vi "StatusPub0MQ.vi"() -> (0 "error":errorcluster)   [LabVIEW 2018]
uses:
  <vilib>/addons/zeromq/zmq_context.lvclass
  <vilib>/addons/zeromq/zmq_socket.lvclass
  <vilib>/addons/zeromq/socket_type.ctl
  Global_Telescopio.vi
  <vilib>/addons/zeromq/zeromq.lvlib
panel:
  out "pulledCommand":string
  out "status":string
  out "time string":string
  in  "panelSstop":bool
  # "TCSPD STATUS PUB\n& \nCOMMAND REP"
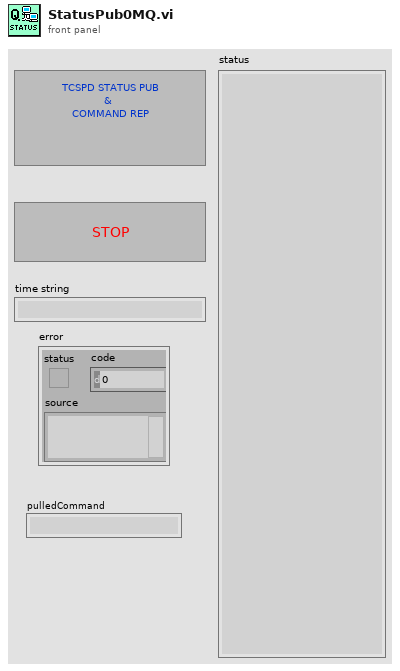
[diagram p1: front panel]
types:
  T1 = typedef "zeromq.lvlib/socket_type.ctl" = enum8{"ZMQ_PAIR", "ZMQ_PUB", "ZMQ_SUB", "ZMQ_REQ", "ZMQ_REP", "ZMQ_DEALER", "ZMQ_ROUTER", "ZMQ_PULL", "ZMQ_PUSH", "ZMQ_XPUB", "ZMQ_XSUB", "ZMQ_STREAM", "ZMQ_SERVER", "ZMQ_CLIENT", "ZMQ_RADIO", "ZMQ_DISH", "ZMQ_GATHER", "ZMQ_SCATTER", "ZMQ_DGRAM"}
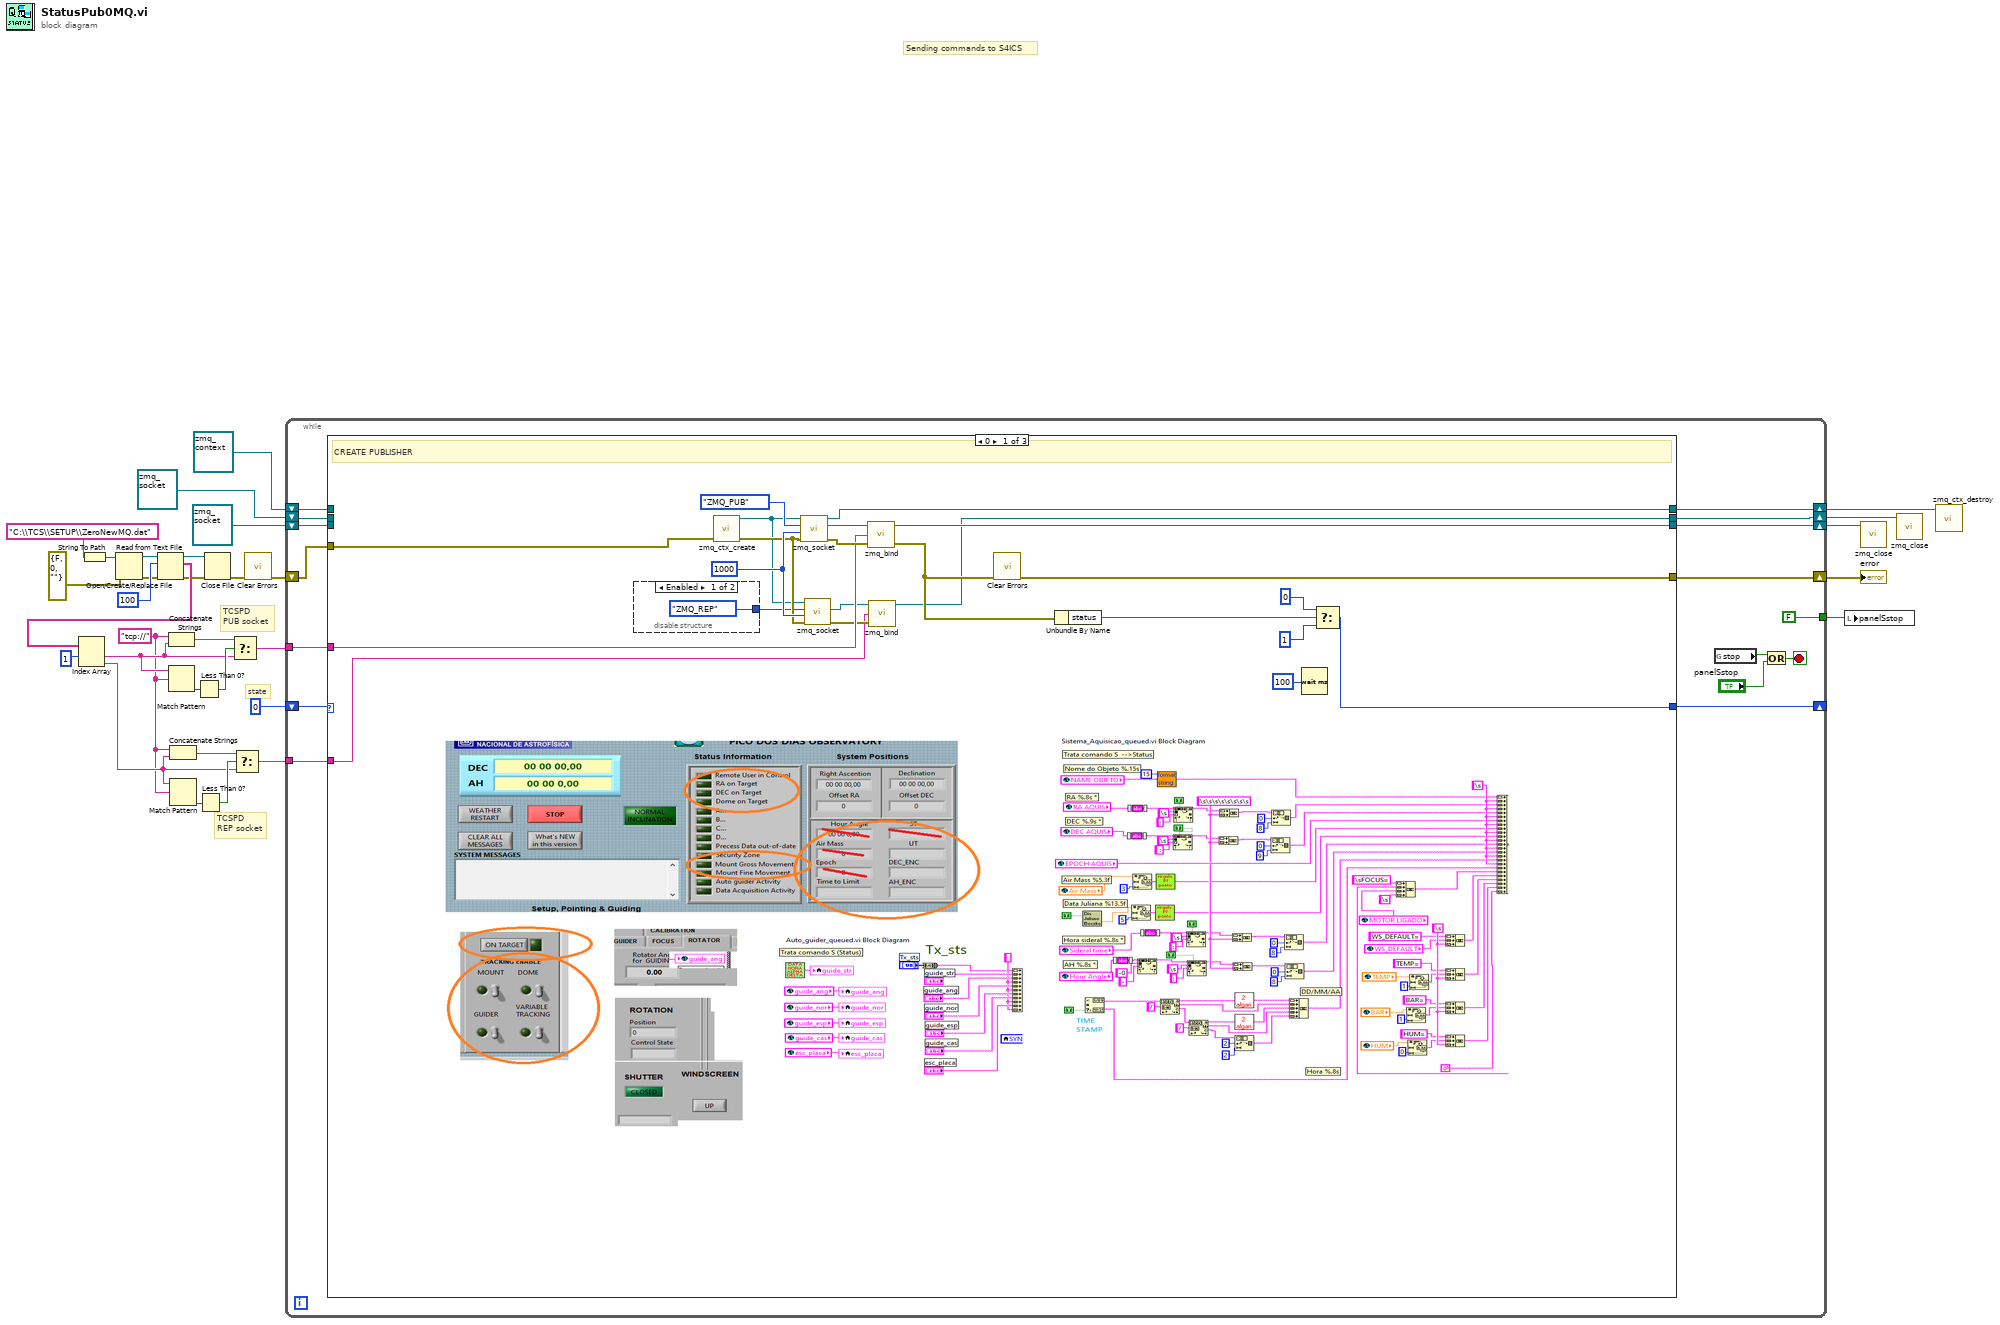
[diagram p0: block diagram]
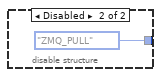
[diagram p2: hidden frame]
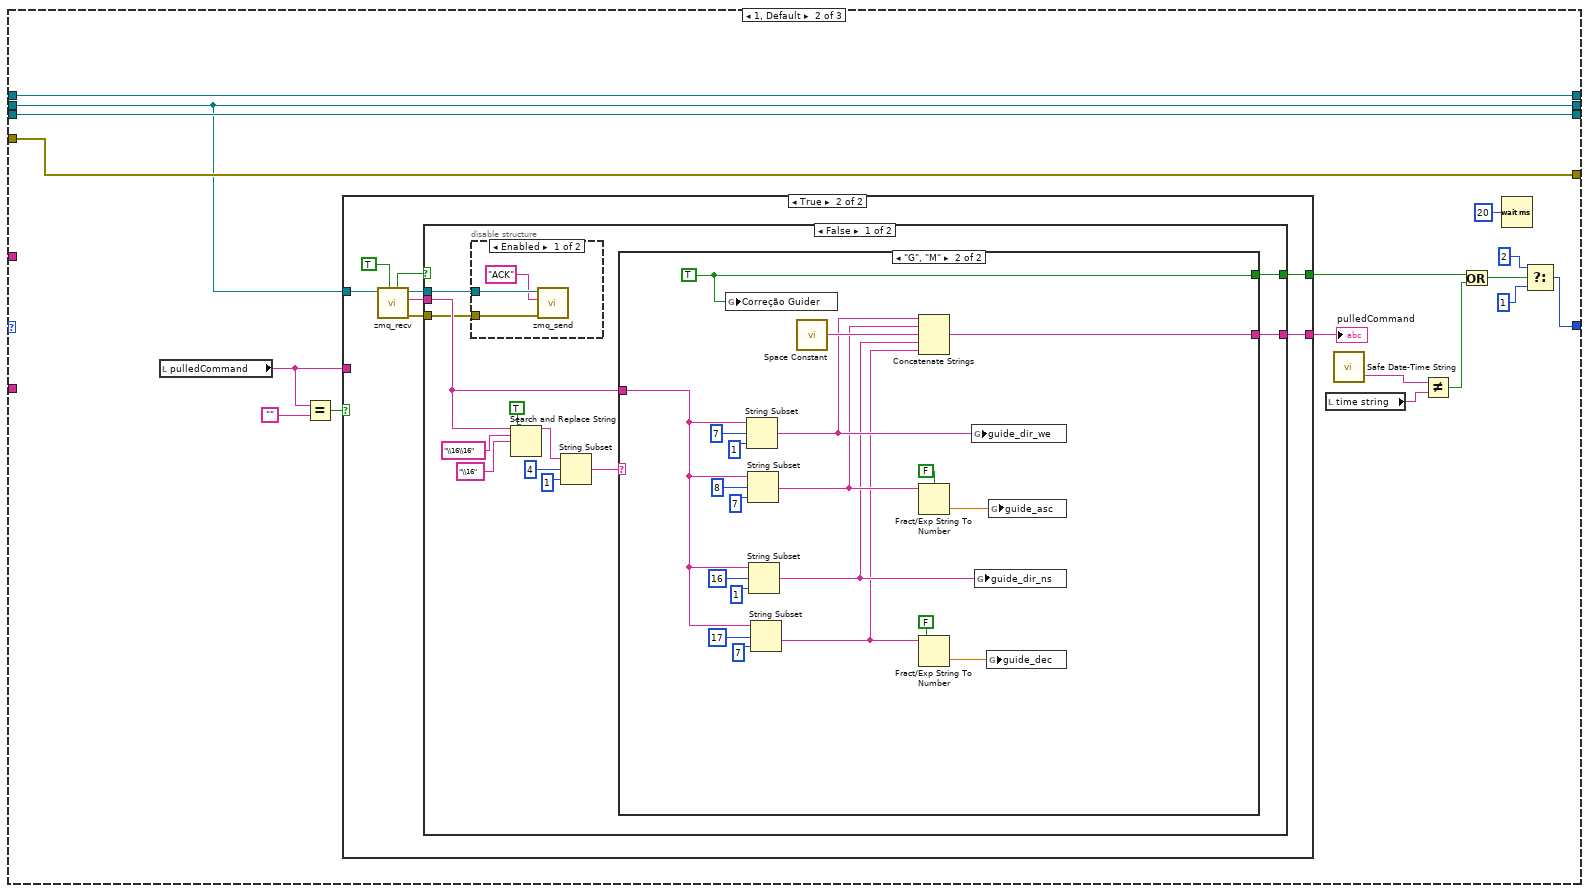
[diagram p3: hidden frame]
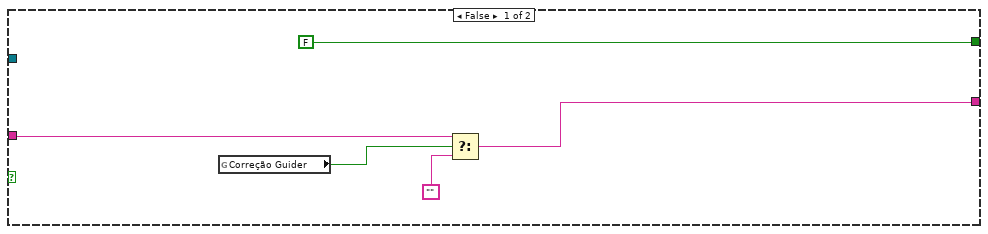
[diagram p4: hidden frame]
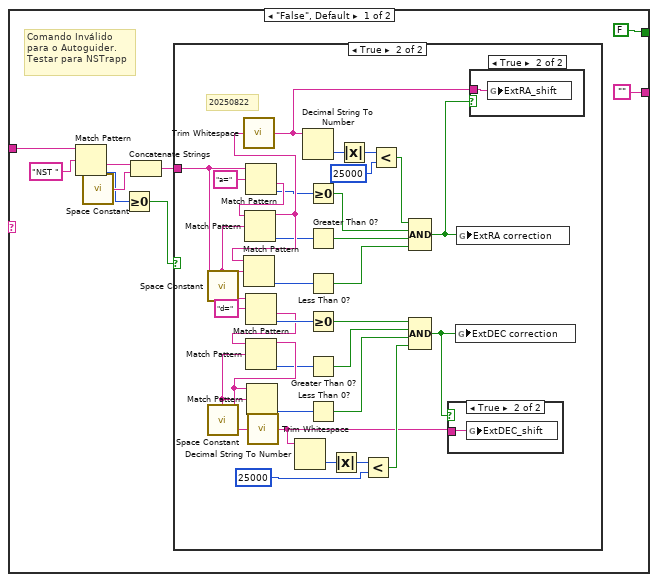
[diagram p6: hidden frame]
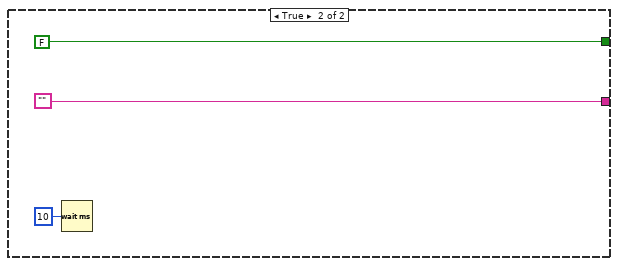
[diagram p10: hidden frame]
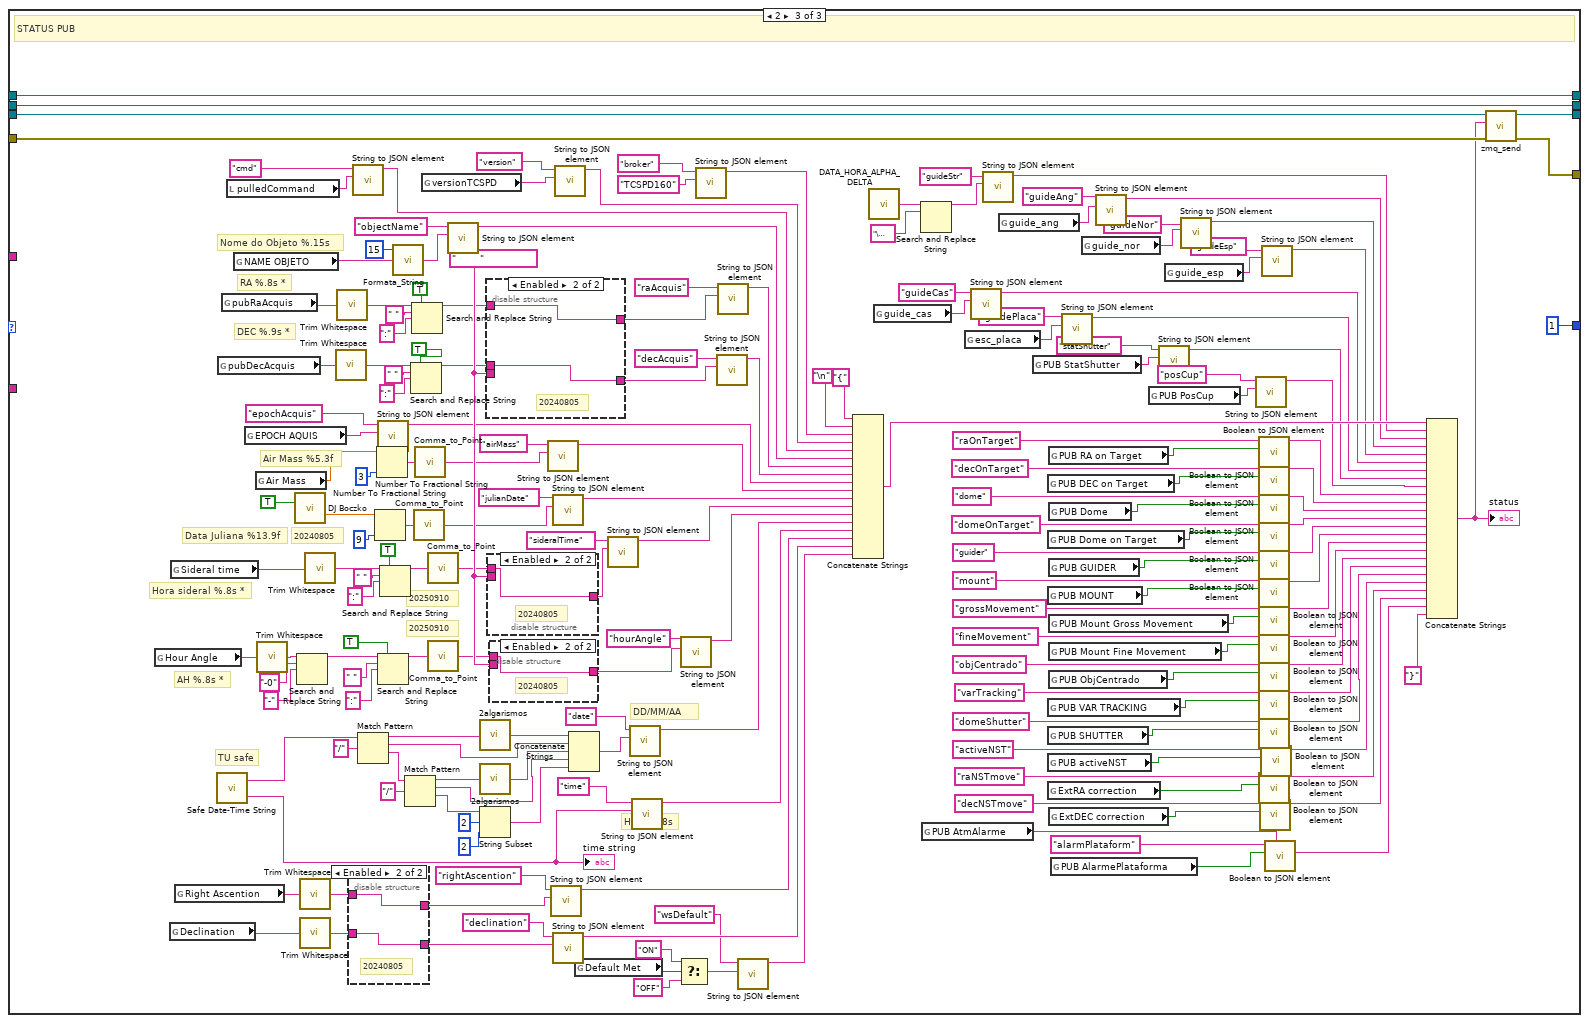
[diagram p11: hidden frame]
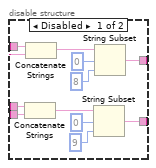
[diagram p12: hidden frame]
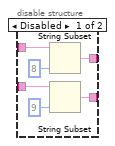
[diagram p13: hidden frame]
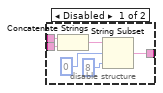
[diagram p14: hidden frame]
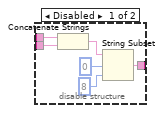
[diagram p15: hidden frame]
diagram:
  w2 = "tcp://"
  # "TCSPD\nREP socket"
  # "TCSPD\nPUB socket"
  # "state"
  # "Sending commands to S4ICS"
  n1 = String To Path(string="C:\\TCS\\SETUP\\ZeroNewMQ.dat") -> (path=w31:path)
  n2 = Open/Create/Replace File(file path (use dialog)=w31, error in=errorcluster {"status"=FALSE, "code"=0, "source"=""}) -> (refnum out=w29:refnum<file>, error out=w22:errorcluster)  [unwired: 4 in, 1 out]
  n3 = Read from Text File(file (use dialog)=w29, count=100, error in=w22) -> (refnum out=w25:refnum<file>, text=w27:string[], error out=w19:errorcluster)  [unwired: 1 in, 1 out]
  n4 = Index Array(array=w27, index #1=1 ("index")) -> (element #1=w11:string, element #2=w3:string)  [unwired: 1 in]
  n5 = Concatenate Strings(w2, w11) -> (w13:string)
  n6 = Match Pattern(string=w11, regular expression=w2) -> (offset past match=w12:i32)  [unwired: 1 in, 3 out]
  n7 = Concatenate Strings(w2, w3) -> (w5:string)
  n8 = Match Pattern(string=w3, regular expression=w2) -> (offset past match=w6:i32)  [unwired: 1 in, 3 out]
  n9 = Less Than 0?(x=w12) -> (x < 0?=w14:bool)
  n10 = Less Than 0?(x=w6) -> (x < 0?=w4:bool)
  n11 = Close File(refnum=w25, error in=w19) -> (error out=w20:errorcluster)  [unwired: 1 out]
  n12 = Select(t=w13, s=w14, f=w11) -> (s? t:f=w10:string)
  n13 = Select(t=w5, s=w4, f=w3) -> (s? t:f=w1:string)
  n14 = call <vilib>:"Clear Errors.vi"("error in (no error)"=w20) -> ("error out"=w18:errorcluster)  [unwired: 5 in, 1 out]
  n15 = while {
    shift-right: [w46] -> _
    shift-left: u16 0 -> [w48]
    tunnel: w10 -> [w44]
    shift-right: [w42] -> w16
    shift-left: refnum<class "zmq_socket.lvclass"> refnum ("socket out") -> [w43]
    shift-right: [w41] -> w21
    shift-left: refnum<class "zmq_context.lvclass"> refnum ("context out") -> [w40]
    tunnel: [FALSE] -> w15
    shift-right: [w37] -> w9
    shift-left: w18 -> [w47]
    shift-right: [w35] -> w7
    shift-left: refnum<class "zmq_socket.lvclass"> refnum ("socket out") -> [w34]
    tunnel: w1 -> [w33]
    stop <- w45 stop-if-true
    n16 = case shown="0" w48 {
      tunnel: w47 -> [w66 w86 w372]
      tunnel: [w68 w87 u16 1] -> w46
      tunnel: w44 -> [w59 _ _]
      tunnel: w43 -> [_ w85 w375]
      tunnel: [w58 w85 w374] -> w42
      tunnel: [w67 w83 w373] -> w41
      tunnel: w40 -> [_ w83 w373]
      tunnel: [w61 w86 w371] -> w37
      tunnel: [w50 w84 w370] -> w35
      tunnel: w34 -> [_ w84 w370]
      tunnel: w33 -> [w49 _ _]
      frame 0 {
        w56 = 1000 ("linger (ms)")
        # "CREATE PUBLISHER"
        n17 = disable-structure shown="Enabled" {
          disable-tunnel: [socket_type."ZMQ_REP" ("socket type") socket_type."ZMQ_PULL" ("socket type")] -> w53
          frame Enabled {
          }
          frame Disabled {
          }
        }
        n18 = call <vilib>:"zmq_ctx_create.vi"("error in"=w66) -> ("error out"=w55:errorcluster, "context out"=w54:refnum<class "zmq_context.lvclass">)  [unwired: 3 in]
        n19 = call <vilib>:"zmq_socket.vi"("error in"=w55, "linger (ms)"=w56, "socket type"=socket_type."ZMQ_PUB", "context in"=w54) -> ("error out"=w63:errorcluster, "socket out"=w64:refnum<class "zmq_socket.lvclass">, "context out"=w67:refnum<class "zmq_context.lvclass">)  [unwired: 1 in]
        n20 = call <vilib>:"zmq_socket.vi"("error in"=w55, "linger (ms)"=w56, "socket type"=w53, "context in"=w54) -> ("error out"=w51:errorcluster, "socket out"=w52:refnum<class "zmq_socket.lvclass">)  [unwired: 1 in, 1 out]
        n21 = call <vilib>:"zmq_bind.vi"("error in"=w63, "endpoint"=w59, "socket in"=w64) -> ("error out"=w60:errorcluster, "socket out"=w58:refnum<class "zmq_socket.lvclass">)  [unwired: 1 in]
        n22 = call <vilib>:"zmq_bind.vi"("error in"=w51, "endpoint"=w49, "socket in"=w52) -> ("socket out"=w50:refnum<class "zmq_socket.lvclass">)  [unwired: 1 in, 1 out]
        n23 = call <vilib>:"Clear Errors.vi"("error in (no error)"=w60) -> ("error out"=w61:errorcluster)  [unwired: 5 in, 1 out]
        n24 = Unbundle By Name(w60) -> ("status"=w57:bool)
        n25 = Wait (ms)(milliseconds to wait=u32 100) -> ()  [unwired: 1 out]
        n26 = Select(t=u16 0, s=w57, f=u16 1) -> (s? t:f=w68:u16)
      }
      frame 1, Default {
        n27 = local read "pulledCommand"() -> (w77:string)
        n28 = Equal?(x=w77, y="") -> (x = y?=w79:bool)
        n29 = case shown="True" w79 {
          tunnel: w84 -> [_ w102]
          tunnel: [w90 w99] -> w74
          tunnel: w77 -> [w92 _]
          tunnel: [FALSE w98] -> w76
          frame False {
            n30 = global read "Global_Telescopio.vi" "Correção Guider"() -> (w93:bool)
            n31 = Select(t=w92, s=w93, f="") -> (s? t:f=w90:string)
          }
          frame True {
            n32 = call <vilib>:"zmq_recv.vi"("no block? (F)"=TRUE, "socket in"=w102) -> ("error out"=w95:errorcluster, "data"=w100:string, "socket out"=w96:refnum<class "zmq_socket.lvclass">, "timeout?"=w97:bool)  [unwired: 3 in, 1 out]
            n33 = case shown="False" w97 {
              tunnel: w100 -> [w107 _]
              tunnel: [w106 ""] -> w99
              tunnel: [w105 FALSE] -> w98
              tunnel: w96 -> [w104 _]
              tunnel: w95 -> [w103 _]
              frame False {
                n34 = disable-structure shown="Enabled" {
                  disable-tunnel: w104 -> [w117 _]
                  disable-tunnel: w103 -> [w116 _]
                  frame Enabled {
                    n35 = call <vilib>:"zmq_send.vi"("error in"=w116, "data"="ACK", "socket in"=w117) -> ()  [unwired: 4 in, 2 out]
                  }
                  frame Disabled {
                  }
                }
                n36 = Search and Replace String(replace all?=TRUE ("replace all? (F)"), input string=w107, search string="\\16\\16", replace string="\\16" ("replace string (\"\")")) -> (result string=w109:string)  [unwired: 4 in, 3 out]
                n37 = String Subset(string=w109, offset (0)=4, length (rest)=1 ("length (rest)")) -> (substring=w108:string)
                n38 = case shown="\"G\", \"M\"" w108 {
                  tunnel: w107 -> [w120 w168]
                  tunnel: ["" w162] -> w106
                  tunnel: [FALSE w169] -> w105
                  frame "False", Default {
                    # "Comando Inválido \npara o Autoguider.\nTestar para NSTrapp"
                    n39 = Match Pattern(string=w120, regular expression="NST ") -> (after substring=w123:string, offset past match=w122:i32)  [unwired: 1 in, 2 out]
                    n40 = call <vilib>:"Space Constant.vi"() -> ("String"=w124:string)
                    n41 = Greater Or Equal To 0?(x=w122) -> (x >= 0?=w118:bool)
                    n42 = Concatenate Strings(w123, w124) -> (w119:string)
                    n43 = case shown="True" w118 {
                      tunnel: w119 -> [_ w131]
                      frame False {
                      }
                      frame True {
                        # "20250822"
                        n44 = call <vilib>:"Space Constant.vi"() -> ("String"=w143:string)
                        n45 = call <vilib>:"Space Constant.vi"() -> ("String"=w148:string)
                        n46 = Match Pattern(string=w131, regular expression="a=") -> (after substring=w135:string, offset past match=w132:i32)  [unwired: 1 in, 2 out]
                        n47 = Match Pattern(string=w135, regular expression=w143) -> (before substring=w142:string, offset past match=w134:i32)  [unwired: 1 in, 2 out]
                        n48 = call <vilib>:"Trim Whitespace.vi"("string"=w142) -> ("trimmed string"=w129:string)  [unwired: 1 in]
                        n49 = Match Pattern(string=w142, regular expression=w143) -> (offset past match=w144:i32)  [unwired: 1 in, 3 out]
                        n50 = Match Pattern(string=w131, regular expression="d=") -> (after substring=w138:string, offset past match=w140:i32)  [unwired: 1 in, 2 out]
                        n51 = Match Pattern(string=w138, regular expression=w148) -> (before substring=w152:string, offset past match=w139:i32)  [unwired: 1 in, 2 out]
                        n52 = Match Pattern(string=w152, regular expression=w148) -> (offset past match=w149:i32)  [unwired: 1 in, 3 out]
                        n53 = call <vilib>:"Trim Whitespace.vi"("string"=w152) -> ("trimmed string"=w130:string)  [unwired: 1 in]
                        n54 = Decimal String To Number(string=w130) -> (number=w151:i32)  [unwired: 2 in, 1 out]
                        n55 = Decimal String To Number(string=w129) -> (number=w157:i32)  [unwired: 2 in, 1 out]
                        n56 = Greater Or Equal To 0?(x=w132) -> (x >= 0?=w137:bool)
                        n57 = Greater Than 0?(x=w134) -> (x > 0?=w136:bool)
                        n58 = Less Than 0?(x=w144) -> (x < 0?=w145:bool)
                        n59 = Greater Or Equal To 0?(x=w140) -> (x >= 0?=w146:bool)
                        n60 = Greater Than 0?(x=w139) -> (x > 0?=w147:bool)
                        n61 = Less Than 0?(x=w149) -> (x < 0?=w150:bool)
                        n62 = Absolute Value(x=w151) -> (abs(x)=w153:i32)
                        n63 = Absolute Value(x=w157) -> (abs(x)=w156:i32)
                        n64 = Less?(x=w153, y=25000 ("abs(x)")) -> (x < y?=w155:bool)
                        n65 = Less?(x=w156, y=25000 ("abs(x)")) -> (x < y?=w159:bool)
                        n66 = Compound Arithmetic op=AND(w159, w137, w136, w145) -> (w127:bool)
                        n67 = Compound Arithmetic op=AND(w146, w147, w150, w155) -> (w128:bool)
                        n68 = case shown="True" w128 {
                          tunnel: w130 -> [_ w161]
                          frame False {
                          }
                          frame True {
                            n69 = global write "Global_Telescopio.vi" "ExtDEC_shift"(w161) -> ()
                          }
                        }
                        n70 = global write "Global_Telescopio.vi" "ExtDEC correction"(w128) -> ()
                        n71 = global write "Global_Telescopio.vi" "ExtRA correction"(w127) -> ()
                        n72 = case shown="True" w127 {
                          tunnel: w129 -> [_ w160]
                          frame False {
                          }
                          frame True {
                            n73 = global write "Global_Telescopio.vi" "ExtRA_shift"(w160) -> ()
                          }
                        }
                      }
                    }
                  }
                  frame "G", "M" {
                    w169 = TRUE ("replace all? (F)")
                    n74 = global write "Global_Telescopio.vi" "Correção Guider"(w169) -> ()
                    n75 = String Subset(string=w168, offset (0)=7, length (rest)=1 ("length (rest)")) -> (substring=w166:string)
                    n76 = String Subset(string=w168, offset (0)=8, length (rest)=7 ("length (rest)")) -> (substring=w165:string)
                    n77 = String Subset(string=w168, offset (0)=16, length (rest)=1 ("length (rest)")) -> (substring=w164:string)
                    n78 = String Subset(string=w168, offset (0)=17, length (rest)=7 ("length (rest)")) -> (substring=w163:string)
                    n79 = call <vilib>:"Space Constant.vi"() -> ("String"=w167:string)
                    n80 = Concatenate Strings(w166, w165, w167, w164, w163) -> (w162:string)
                    n81 = Fract/Exp String To Number(use system decimal point (T)=FALSE, string=w165) -> (number=w180:dbl)  [unwired: 2 in, 1 out]
                    n82 = Fract/Exp String To Number(use system decimal point (T)=FALSE, string=w163) -> (number=w181:dbl)  [unwired: 2 in, 1 out]
                    n83 = global write "Global_Telescopio.vi" "guide_dir_we"(w166) -> ()
                    n84 = global write "Global_Telescopio.vi" "guide_dir_ns"(w164) -> ()
                    n85 = global write "Global_Telescopio.vi" "guide_dec"(w181) -> ()
                    n86 = global write "Global_Telescopio.vi" "guide_asc"(w180) -> ()
                  }
                }
              }
              frame True {
                n87 = Wait (ms)(milliseconds to wait=u32 10) -> ()  [unwired: 1 out]
              }
            }
          }
        }
        "pulledCommand" <- w74
        n88 = local read "time string"() -> (w80:string)
        n89 = call "Safe Date-Time String.vi"() -> ("Safe time string"=w73:string)  [unwired: 3 in, 1 out]
        n90 = Not Equal?(x=w73, y=w80) -> (x != y?=w81:bool)
        n91 = Or(x=w76, y=w81) -> (x .or. y?=w82:bool)
        n92 = Wait (ms)(milliseconds to wait=u32 20) -> ()  [unwired: 1 out]
        n93 = Select(t=u16 2, s=w82, f=u16 1) -> (s? t:f=w87:u16)
      }
      frame 2 {
        w346 = "        " ("string")
        # "20250910"
        # "20250910"
        # "TU safe"
        # "20240805"
        # "Hora %.8s"
        # "DD/MM/AA"
        # "AH %.8s *"
        # "Hora sideral %.8s *"
        # "Data Juliana %13.9f"
        # "Air Mass %5.3f"
        # "DEC %.9s *"
        # "RA %.8s *"
        # "Nome do Objeto %.15s"
        # "STATUS PUB"
        n94 = global read "Global_Telescopio.vi" "Hour Angle"() -> (w369:string)
        n95 = global read "Global_Telescopio.vi" "Declination"() -> (w236:string)
        n96 = global read "Global_Telescopio.vi" "Sideral time"() -> (w342:string)
        n97 = global read "Global_Telescopio.vi" "Right Ascention"() -> (w234:string)
        n98 = call "Safe Date-Time String.vi"() -> ("Safe time string"=w202:string, "Safe date string"=w201:string)  [unwired: 3 in]
        "time string" <- w202
        n99 = global read "Global_Telescopio.vi" "pubDecAcquis"() -> (w332:string)
        n100 = global read "Global_Telescopio.vi" "pubRaAcquis"() -> (w322:string)
        n101 = local read "pulledCommand"() -> (w219:string)
        n102 = global read "Global_Telescopio.vi" "NAME OBJETO"() -> (w363:string)
        n103 = global read "Global_Telescopio.vi" "EPOCH AQUIS"() -> (w311:string)
        n104 = global read "Global_Telescopio.vi" "Air Mass"() -> (w362:dbl)
        n105 = call <vilib>:"Trim Whitespace.vi"("string"=w369) -> ("trimmed string"=w368:string)  [unwired: 1 in]
        n106 = call "DJ Boczko.vi"("TRUE = Hora Local\nFALSE = UT"=TRUE ("TRUE = Hora Local\nFALSE = UT")) -> ("Dia Juliano"=w337:dbl)  [unwired: 6 in, 8 out]
        n107 = Search and Replace String(input string=w368, search string="-0", replace string="-" ("replace string (\"\")")) -> (result string=w367:string)  [unwired: 5 in, 3 out]
        n108 = call <vilib>:"Trim Whitespace.vi"("string"=w234) -> ("trimmed string"=w233:string)  [unwired: 1 in]
        n109 = call <vilib>:"Trim Whitespace.vi"("string"=w236) -> ("trimmed string"=w235:string)  [unwired: 1 in]
        n110 = call <vilib>:"Trim Whitespace.vi"("string"=w342) -> ("trimmed string"=w341:string)  [unwired: 1 in]
        n111 = call <vilib>:"Trim Whitespace.vi"("string"=w332) -> ("trimmed string"=w331:string)  [unwired: 1 in]
        n112 = call <vilib>:"Trim Whitespace.vi"("string"=w322) -> ("trimmed string"=w323:string)  [unwired: 1 in]
        n113 = disable-structure shown="Enabled" {
          disable-tunnel: w235 -> [w395 w396]
          disable-tunnel: w233 -> [w393 w397]
          disable-tunnel: [w392 w397] -> w227
          disable-tunnel: [w391 w396] -> w226
          frame Disabled {
            n114 = String Subset(string=w393, length (rest)=8 ("length (rest)")) -> (substring=w392:string)  [unwired: 1 in]
            n115 = String Subset(string=w395, length (rest)=9 ("length (rest)")) -> (substring=w391:string)  [unwired: 1 in]
          }
          frame Enabled {
            # "20240805"
          }
        }
        n116 = call "String to JSON element.vi"("value"=w219, "keyword"="cmd") -> ("JSON element"=w214:string)  [unwired: 8 in, 1 out]
        n117 = Match Pattern(string=w201, regular expression="/") -> (before substring=w350:string, match substring=w356:string, after substring=w349:string)  [unwired: 1 in, 1 out]
        n118 = Number To Fractional String(number=w337, precision (6)=i16 9) -> (F-format string=w338:string)  [unwired: 2 in]
        n119 = Number To Fractional String(number=w362, precision (6)=i16 3) -> (F-format string=w335:string)  [unwired: 2 in]
        n120 = call "String to JSON element.vi"("value"=w311, "keyword"="epochAcquis") -> ("JSON element"=w310:string)  [unwired: 8 in, 1 out]
        n121 = Search and Replace String(replace all?=TRUE ("replace all? (F)"), input string=w367, search string=" ", replace string=":" ("replace string (\"\")")) -> (result string=w195:string)  [unwired: 4 in, 3 out]
        n122 = Search and Replace String(replace all?=TRUE ("replace all? (F)"), input string=w341, search string=" ", replace string=":" ("replace string (\"\")")) -> (result string=w197:string)  [unwired: 4 in, 3 out]
        n123 = call "Formata_String.vi"("entrada"=w363, "Num de Caracteres"=15) -> ("saida"=w320:string)  [unwired: 3 in]
        n124 = Match Pattern(string=w349, regular expression="/") -> (before substring=w351:string, match substring=w358:string, after substring=w352:string)  [unwired: 1 in, 1 out]
        n125 = Search and Replace String(replace all?=TRUE ("replace all? (F)"), input string=w331, search string=" ", replace string=":" ("replace string (\"\")")) -> (result string=w328:string)  [unwired: 4 in, 3 out]
        n126 = Search and Replace String(replace all?=TRUE ("replace all? (F)"), input string=w323, search string=" ", replace string=":" ("replace string (\"\")")) -> (result string=w327:string)  [unwired: 4 in, 3 out]
        n127 = call "Comma_to_Point.vi"("Lat_A"=w338) -> ("Saída"=w199:string)
        n128 = call "Comma_to_Point.vi"("Lat_A"=w335) -> ("Saída"=w309:string)
        n129 = global read "Global_Telescopio.vi" "versionTCSPD"() -> (w194:string)
        n130 = call "Comma_to_Point.vi"("Lat_A"=w197) -> ("Saída"=w198:string)
        n131 = call "Comma_to_Point.vi"("Lat_A"=w195) -> ("Saída"=w196:string)
        n132 = call "String to JSON element.vi"("value"=w320, "keyword"="objectName") -> ("JSON element"=w319:string)  [unwired: 8 in, 1 out]
        n133 = call "2algarismos.vi"("entrada"=w350) -> ("saida"=w355:string)
        n134 = call "2algarismos.vi"("entrada"=w351) -> ("saida"=w357:string)
        n135 = String Subset(string=w352, offset (0)=2, length (rest)=2 ("length (rest)")) -> (substring=w359:string)
        n136 = disable-structure shown="Enabled" {
          disable-tunnel: w346 -> [w387 _]
          disable-tunnel: w328 -> [w384 w389]
          disable-tunnel: w327 -> [w381 w388]
          disable-tunnel: [w378 w388] -> w318
          disable-tunnel: [w377 w389] -> w315
          frame Disabled {
            n137 = Concatenate Strings(w384, w387) -> (w383:string)
            n138 = Concatenate Strings(w381, w387) -> (w382:string)
            n139 = String Subset(string=w383, offset (0)=0, length (rest)=9 ("length (rest)")) -> (substring=w377:string)
            n140 = String Subset(string=w382, offset (0)=0, length (rest)=8 ("length (rest)")) -> (substring=w378:string)
          }
          frame Enabled {
            # "20240805"
          }
        }
        n141 = disable-structure shown="Enabled" {
          disable-tunnel: w346 -> [w410 _]
          disable-tunnel: w198 -> [w407 w411]
          disable-tunnel: [w405 w411] -> w303
          frame Disabled {
            n142 = Concatenate Strings(w407, w410) -> (w406:string)
            n143 = String Subset(string=w406, offset (0)=0, length (rest)=8 ("length (rest)")) -> (substring=w405:string)
          }
          frame Enabled {
            # "20240805"
          }
        }
        n144 = disable-structure shown="Enabled" {
          disable-tunnel: w346 -> [w403 _]
          disable-tunnel: w196 -> [w401 w404]
          disable-tunnel: [w398 w404] -> w300
          frame Disabled {
            n145 = Concatenate Strings(w401, w403) -> (w402:string)
            n146 = String Subset(string=w402, offset (0)=0, length (rest)=8 ("length (rest)")) -> (substring=w398:string)
          }
          frame Enabled {
            # "20240805"
          }
        }
        n147 = call "String to JSON element.vi"("value"=w309, "keyword"="airMass") -> ("JSON element"=w307:string)  [unwired: 8 in, 1 out]
        n148 = call "String to JSON element.vi"("value"=w227, "keyword"="rightAscention") -> ("JSON element"=w225:string)  [unwired: 8 in, 1 out]
        n149 = call "String to JSON element.vi"("value"=w199, "keyword"="julianDate") -> ("JSON element"=w305:string)  [unwired: 8 in, 1 out]
        n150 = call "String to JSON element.vi"("value"=w226, "keyword"="declination") -> ("JSON element"=w224:string)  [unwired: 8 in, 1 out]
        n151 = call "String to JSON element.vi"("value"=w194, "keyword"="version") -> ("JSON element"=w215:string)  [unwired: 8 in, 1 out]
        n152 = Concatenate Strings(w355, w356, w357, w358, w359) -> (w297:string)
        n153 = global read "Global_Telescopio.vi" "Default Met"() -> (w210:bool)
        n154 = call "String to JSON element.vi"("value"=w303, "keyword"="sideralTime") -> ("JSON element"=w302:string)  [unwired: 8 in, 1 out]
        n155 = call "String to JSON element.vi"("value"=w297, "keyword"="date") -> ("JSON element"=w296:string)  [unwired: 8 in, 1 out]
        n156 = call "String to JSON element.vi"("value"=w202, "keyword"="time") -> ("JSON element"=w294:string)  [unwired: 8 in, 1 out]
        n157 = Select(t="ON", s=w210, f="OFF") -> (s? t:f=w208:string)
        n158 = call "String to JSON element.vi"("value"=w300, "keyword"="hourAngle") -> ("JSON element"=w299:string)  [unwired: 8 in, 1 out]
        n159 = call "String to JSON element.vi"("value"="TCSPD160", "keyword"="broker") -> ("JSON element"=w216:string)  [unwired: 8 in, 1 out]
        n160 = call "String to JSON element.vi"("value"=w315, "keyword"="decAcquis") -> ("JSON element"=w313:string)  [unwired: 8 in, 1 out]
        n161 = call "String to JSON element.vi"("value"=w318, "keyword"="raAcquis") -> ("JSON element"=w316:string)  [unwired: 8 in, 1 out]
        n162 = call "String to JSON element.vi"("value"=w208, "keyword"="wsDefault") -> ("JSON element"=w212:string)  [unwired: 8 in, 1 out]
        n163 = Concatenate Strings("{", "\n", w216, w215, w214, w319, w316, w313, w310, w307, w305, w302, w299, w296, w294, w225, w224, w212) -> (w256:string)
        n164 = call "DATA_HORA_ALPHA_DELTA.vi"() -> ("SAIDA"=w232:string)  [unwired: 2 in]
        n165 = global read "Global_Telescopio.vi" "guide_cas"() -> (w285:string)
        n166 = Search and Replace String(input string=w232, search string="\u0000") -> (result string=w230:string)  [unwired: 6 in, 3 out]
        n167 = global read "Global_Telescopio.vi" "PUB AtmAlarme"() -> (w187:string)
        n168 = global read "Global_Telescopio.vi" "esc_placa"() -> (w283:string)
        n169 = call "String to JSON element.vi"("value"=w285, "keyword"="guideCas") -> ("JSON element"=w251:string)  [unwired: 8 in, 1 out]
        n170 = call "String to JSON element.vi"("value"=w230, "keyword"="guideStr") -> ("JSON element"=w255:string)  [unwired: 8 in, 1 out]
        n171 = global read "Global_Telescopio.vi" "guide_ang"() -> (w291:string)
        n172 = global read "Global_Telescopio.vi" "PUB StatShutter"() -> (w260:string)
        n173 = global read "Global_Telescopio.vi" "PUB DEC on Target"() -> (w271:bool)
        n174 = global read "Global_Telescopio.vi" "PUB Dome on Target"() -> (w269:bool)
        n175 = global read "Global_Telescopio.vi" "PUB MOUNT"() -> (w267:bool)
        n176 = global read "Global_Telescopio.vi" "PUB VAR TRACKING"() -> (w263:bool)
        n177 = global read "Global_Telescopio.vi" "PUB SHUTTER"() -> (w261:bool)
        n178 = global read "Global_Telescopio.vi" "PUB activeNST"() -> (w191:bool)
        n179 = global read "Global_Telescopio.vi" "ExtRA correction"() -> (w190:bool)
        n180 = global read "Global_Telescopio.vi" "PUB RA on Target"() -> (w272:bool)
        n181 = global read "Global_Telescopio.vi" "PUB Dome"() -> (w270:bool)
        n182 = global read "Global_Telescopio.vi" "PUB GUIDER"() -> (w268:bool)
        n183 = global read "Global_Telescopio.vi" "PUB Mount Gross Movement"() -> (w266:bool)
        n184 = global read "Global_Telescopio.vi" "PUB Mount Fine Movement"() -> (w265:bool)
        n185 = global read "Global_Telescopio.vi" "PUB ObjCentrado"() -> (w264:bool)
        n186 = global read "Global_Telescopio.vi" "ExtDEC correction"() -> (w189:bool)
        n187 = global read "Global_Telescopio.vi" "PUB AlarmePlataforma"() -> (w188:bool)
        n188 = call "String to JSON element.vi"("value"=w283, "keyword"="guidePlaca") -> ("JSON element"=w250:string)  [unwired: 8 in, 1 out]
        n189 = global read "Global_Telescopio.vi" "guide_nor"() -> (w289:string)
        n190 = call "String to JSON element.vi"("value"=w291, "keyword"="guideAng") -> ("JSON element"=w254:string)  [unwired: 8 in, 1 out]
        n191 = global read "Global_Telescopio.vi" "PUB PosCup"() -> (w259:string)
        n192 = call "String to JSON element.vi"("value"=w260, "keyword"="statShutter") -> ("JSON element"=w249:string)  [unwired: 8 in, 1 out]
        n193 = global read "Global_Telescopio.vi" "guide_esp"() -> (w287:string)
        n194 = call "String to JSON element.vi"("value"=w289, "keyword"="guideNor") -> ("JSON element"=w253:string)  [unwired: 8 in, 1 out]
        n195 = call "String to JSON element.vi"("value"=w259, "keyword"="posCup") -> ("JSON element"=w248:string)  [unwired: 8 in, 1 out]
        n196 = call "Boolean to JSON element.vi"("boolean"=w272, "keyword"="raOnTarget") -> ("JSON element"=w247:string)  [unwired: 8 in, 1 out]
        n197 = call "Boolean to JSON element.vi"("boolean"=w271, "keyword"="decOnTarget") -> ("JSON element"=w246:string)  [unwired: 8 in, 1 out]
        n198 = call "Boolean to JSON element.vi"("boolean"=w270, "keyword"="dome") -> ("JSON element"=w245:string)  [unwired: 8 in, 1 out]
        n199 = call "Boolean to JSON element.vi"("boolean"=w269, "keyword"="domeOnTarget") -> ("JSON element"=w244:string)  [unwired: 8 in, 1 out]
        n200 = call "Boolean to JSON element.vi"("boolean"=w268, "keyword"="guider") -> ("JSON element"=w243:string)  [unwired: 8 in, 1 out]
        n201 = call "Boolean to JSON element.vi"("boolean"=w267, "keyword"="mount") -> ("JSON element"=w242:string)  [unwired: 8 in, 1 out]
        n202 = call "Boolean to JSON element.vi"("boolean"=w266, "keyword"="grossMovement") -> ("JSON element"=w241:string)  [unwired: 8 in, 1 out]
        n203 = call "Boolean to JSON element.vi"("boolean"=w265, "keyword"="fineMovement") -> ("JSON element"=w240:string)  [unwired: 8 in, 1 out]
        n204 = call "Boolean to JSON element.vi"("boolean"=w264, "keyword"="objCentrado") -> ("JSON element"=w239:string)  [unwired: 8 in, 1 out]
        n205 = call "Boolean to JSON element.vi"("boolean"=w263, "keyword"="varTracking") -> ("JSON element"=w238:string)  [unwired: 8 in, 1 out]
        n206 = call "Boolean to JSON element.vi"("boolean"=w261, "keyword"="domeShutter") -> ("JSON element"=w200:string)  [unwired: 8 in, 1 out]
        n207 = call "Boolean to JSON element.vi"("boolean"=w190, "keyword"="raNSTmove") -> ("JSON element"=w203:string)  [unwired: 8 in, 1 out]
        n208 = call "Boolean to JSON element.vi"("boolean"=w189, "keyword"="decNSTmove") -> ("JSON element"=w193:string)  [unwired: 8 in, 1 out]
        n209 = call "Boolean to JSON element.vi"("boolean"=w191, "keyword"="activeNST") -> ("JSON element"=w204:string)  [unwired: 8 in, 1 out]
        n210 = call "String to JSON element.vi"("value"=w287, "keyword"="guideEsp") -> ("JSON element"=w252:string)  [unwired: 8 in, 1 out]
        n211 = call "Boolean to JSON element.vi"("prefix"=w187, "boolean"=w188, "keyword"="alarmPlataform") -> ("JSON last element"=w186:string)  [unwired: 7 in, 1 out]
        n212 = Concatenate Strings(w256, w255, w254, w253, w252, w251, w250, w249, w248, w247, w246, w245, w244, w243, w242, w241, w240, w239, w238, w200, w204, w203, w193, w186, "}") -> (w237:string)
        "status" <- w237
        n213 = call <vilib>:"zmq_send.vi"("error in"=w372, "data"=w237, "socket in"=w375) -> ("error out"=w371:errorcluster, "socket out"=w374:refnum<class "zmq_socket.lvclass">)  [unwired: 4 in]
      }
    }
    n214 = global read "Global_Telescopio.vi" "stop"() -> (w36:bool)
    n215 = Or(x=w36, y="panelSstop") -> (x .or. y?=w45:bool)
  }
  "error" <- w9
  n216 = local write "panelSstop"(w15) -> ()
  n217 = call <vilib>:"zmq_close.vi"("socket"=w16) -> ()  [unwired: 4 in, 1 out]
  n218 = call <vilib>:"zmq_close.vi"("socket"=w7) -> ()  [unwired: 4 in, 1 out]
  n219 = call <vilib>:"zmq_ctx_destroy.vi"("context in"=w21) -> ()  [unwired: 4 in, 1 out]
